vi "IOMAC5000.vi"(0 "VISA  IN":refnum<visa-resource-name>, 2 "Dwell Time (ms)":u32(knob)=75 scale=0.0..100.0, 5 "Communication Port":i32(ring) items=["COM1", "USB"], 7 "Command (to ctlr)":string, 11 "error in":errorcluster) -> (4 "VISA OUT":refnum<visa-resource-name>, 6 "Communication Port Out":i32(ring) items=["COM1", "USB"], 8 "Raw Response":string, 15 "error out":errorcluster)   [LabVIEW 2022 SP3, in "Stage Controller.lvlib"]
doc: "SubVI for sending commands to the MAC5000 and receiving responses from the MAC5000."
uses:
  Stage Controller.lvlib
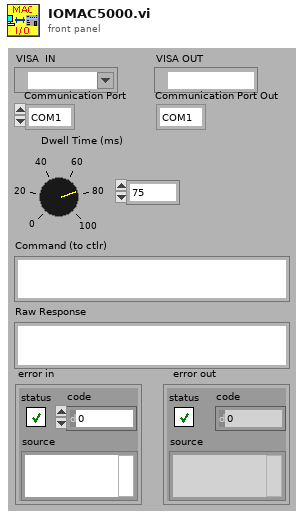
[diagram p1: front panel]
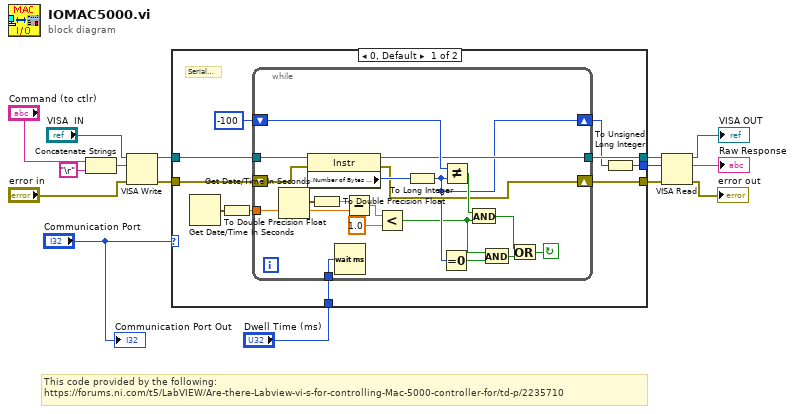
[diagram p0: block diagram]
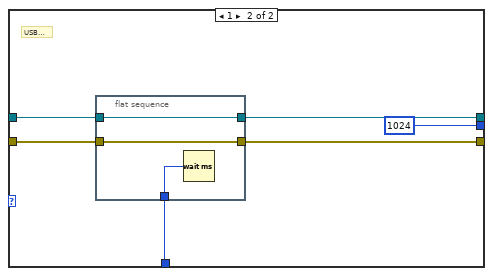
[diagram p2: hidden frame]
diagram:
  # "This code provided by the following:\nhttps://forums.ni.com/t5/LabVIEW/Are-there-Labview-vi-s-for-controlling-Mac-5000-controller-for/td-p/2235710"
  n1 = Concatenate Strings("Command (to ctlr)", "\r") -> (w1:string)
  n2 = VISA Write(VISA resource name="VISA  IN", write buffer=w1, error in (no error)="error in") -> (VISA resource name out=w14:refnum<visa-resource-name>, error out=w12:errorcluster)  [unwired: 1 out]
  n3 = case shown="0, Default" "Communication Port" {
    tunnel: w14 -> [w25 w50]
    tunnel: w12 -> [w23 w47]
    tunnel: [w20 w49] -> w11
    tunnel: [w19 w46] -> w10
    tunnel: [w18 u32 1024] -> w9
    tunnel: "Dwell Time (ms)" -> [w17 w45]
    frame 0, Default {
      # "Serial Port"
      n4 = Get Date/Time In Seconds() -> (seconds since 1Jan1904=w22:timestamp)
      n5 = To Double Precision Float(number=w22) -> (double precision float=w21:dbl)
      n6 = while {
        shift-right: [w33] -> w16
        shift-left: -100 -> [w42]
        tunnel: w25 -> [w44]
        shift-right: [w35] -> w19
        shift-left: w23 -> [w41]
        tunnel: w21 -> [w29]
        tunnel: [w39] -> w20
        tunnel: w17 -> [w34]
        stop <- w31 continue-if-true
        n7 = Get Date/Time In Seconds() -> (seconds since 1Jan1904=w40:timestamp)
        n8 = property class="Instr"(reference=w44, error in=w41) -> (reference out=w39:refnum<visa-resource-name>, error out=w35:errorcluster, "Serial Settings:Number of Bytes at Serial Port"=w43:u32)
        n9 = To Double Precision Float(number=w40) -> (double precision float=w30:dbl)
        n10 = Wait (ms)(milliseconds to wait=w34) -> ()  [unwired: 1 out]
        n11 = Subtract(x=w30, y=w29) -> (x-y=w38:dbl)
        n12 = Less?(x=w38, y=1.0) -> (x < y?=w26:bool)
        n13 = To Long Integer(number=w43) -> (32bit integer=w33:i32)
        n14 = Equal To 0?(x=w33) -> (x = 0?=w27:bool)
        n15 = Not Equal?(x=w42, y=w33) -> (x != y?=w36:bool)
        n16 = And(x=w36, y=w26) -> (x .and. y?=w32:bool)
        n17 = And(x=w26, y=w27) -> (x .and. y?=w28:bool)
        n18 = Or(x=w32, y=w28) -> (x .or. y?=w31:bool)
      }
      n19 = To Unsigned Long Integer(number=w16) -> (unsigned 32bit integer=w18:u32)
    }
    frame 1 {
      # "USB Port"
      n20 = flat-sequence {
        tunnel: w50 -> [w53]
        tunnel: [w53] -> w49
        tunnel: w47 -> [w52]
        tunnel: [w52] -> w46
        tunnel: w45 -> [w51]
        frame #0 {
          n21 = Wait (ms)(milliseconds to wait=w51) -> ()  [unwired: 1 out]
        }
      }
    }
  }
  n22 = VISA Read(VISA resource name=w11, byte count=w9, error in (no error)=w10) -> (VISA resource name out=→"VISA OUT":refnum<visa-resource-name>, read buffer=→"Raw Response":string, error out=→"error out":errorcluster)  [unwired: 1 out]
  "Communication Port Out" <- "Communication Port"
